vi "Add Port (MIL 1553).vi"(8 "error in":errorcluster, 10 "port number":u16, 11 "Ballard MIL-STD 1553 custom device in":T1 format="%.0x") -> (0 "error out":errorcluster, 2 "port":T1 format="%.0x", 3 "Ballard MIL-STD 1553 custom device out":T1 format="%.0x")   [LabVIEW 2020, in "Ballard MIL-STD-1553 Scripting.lvlib"]
uses:
  Ballard MIL-STD-1553 Scripting.lvlib
  <vilib>/NI VeriStand/Custom Device API/Custom Device Item Ref.ctl
  Constants.vi
  <vilib>/NI VeriStand/Custom Device API/Custom Device API.lvlib
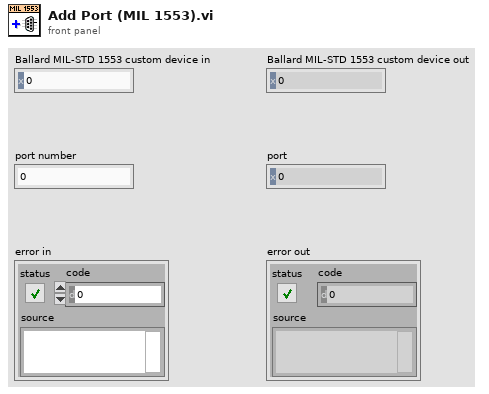
[diagram p1: front panel]
types:
  T1 = typedef "Custom Device API.lvlib/Custom Device Item Ref.ctl" = u64
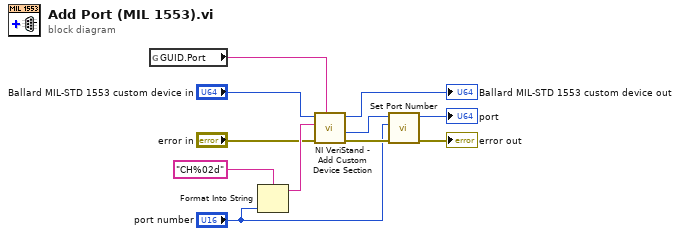
[diagram p0: block diagram]
diagram:
  n1 = global read "Constants.vi" "GUID.Port"() -> (w1:string)
  n2 = Format Into String(format string="CH%02d", "port number") -> (resulting string=w10:string)  [unwired: 2 in, 1 out]
  n3 = call <vilib>:"NI VeriStand - Add Custom Device Section.vi"("GUID (Default Section)"=w1, "error in (no error)"="error in", "Section Name"=w10, "Parent Ref in"="Ballard MIL-STD 1553 custom device in") -> ("error out"=w5:errorcluster, "Section Ptr"=w6:T1, "Parent Ref out"=→"Ballard MIL-STD 1553 custom device out":T1)  [unwired: 4 in, 1 out]
  n4 = call "Set Port Number.vi"("error in"=w5, "port number"="port number", "port in"=w6) -> ("error out"=→"error out":errorcluster, "port out"=→"port":T1)  [unwired: 7 in]
